vi "turret_theta.vi"(9 "Target y (Deg)":dbl(slide) scale=-20.5..20.5, 10 "Target x (deg)":dbl(slide) scale=-27.0..27.0) -> (1 "Theta":dbl, 2 "Target Distance (in)":dbl(slide) scale=0.0..350.0)   [LabVIEW 2020]
uses:
  <vilib>/Analysis/coordinate.llb/2D Cartesian Coordinate Rotation (Scalar).vi
  <vilib>/Analysis/NI_AALPro.lvlib
  TitanLib/Lib/TitanLib.lvlib
panel:
  out "Graph":cluster{"X":dbl, "Y":dbl}[](graph)
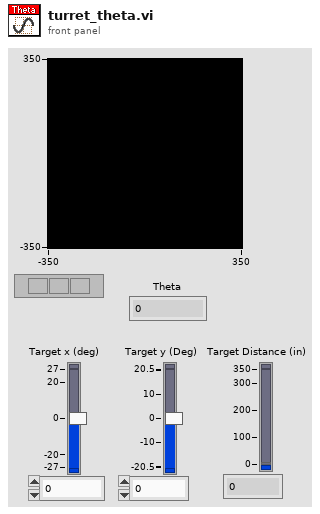
[diagram p1: front panel]
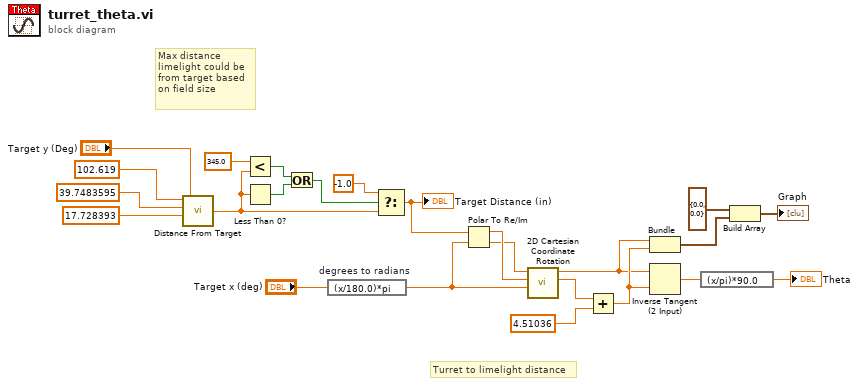
[diagram p0: block diagram]
diagram:
  # "Turret to limelight distance"
  # "Max distance\nlimelight could be\nfrom target based\non field size"
  n1 = call "Distance From Target.vi"("Target Angle (Deg)"="Target y (Deg)", "Camera Angle (Deg)"=17.728393, "Camera Height (in)"=39.7483595, "Target Height (in)"=102.619) -> ("Distance (in)"=w7:dbl)
  n2 = Less?(x=345.0, y=w7) -> (x < y?=w5:bool)
  n3 = Less Than 0?(x=w7) -> (x < 0?=w6:bool)
  n4 = Or(x=w5, y=w6) -> (x .or. y?=w4:bool)
  n5 = expression code="(x/180.0)*pi" "degrees to radians"("Target x (deg)") -> (w20:dbl)
  n6 = Select(t=-1.0, s=w4, f=w7) -> (s? t:f=w10:dbl)
  "Target Distance (in)" <- w10
  n7 = Polar To Re/Im(2:w20, 3:w10) -> (0:w8:dbl, 1:w9:dbl)
  n8 = call-poly <vilib>:"2D Cartesian Coordinate Rotation.vi"("theta"=w20, "y"=w9, "x"=w8) -> ("y out"=w17:dbl, "x out"=w2:dbl)  [unwired: 6 in, 1 out]
  n9 = Add(x=w17, y=4.51036) -> (x+y=w3:dbl)
  n10 = Bundle("x out"=w2, w3) -> (w18:cluster{"x out":dbl, dbl})  [unwired: 1 in]
  n11 = Inverse Tangent (2 Input)(1:w3, 2:w2) -> (0:w19:dbl)
  n12 = expression code="(x/pi)*90.0" ("radians to degrees")(w19) -> (→"Theta":dbl)
  n13 = Build Array(cluster{dbl, dbl} {0.0, 0.0} ("element"), w18) -> (→"Graph":cluster{"x out":dbl, dbl}[])
